vi "Configure ExecutionView Manager.vi"(8 "error in":errorcluster) -> (0 "error out":errorcluster)   [LabVIEW 2025, in "Config Tool.lvlib"]
doc: "This VI configures the Connections and Commands for the ExecutionView Manager."
uses:
  Control Globals.vi
  Config Tool.lvlib
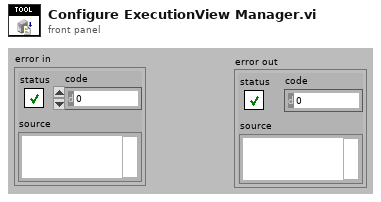
[diagram p1: front panel]
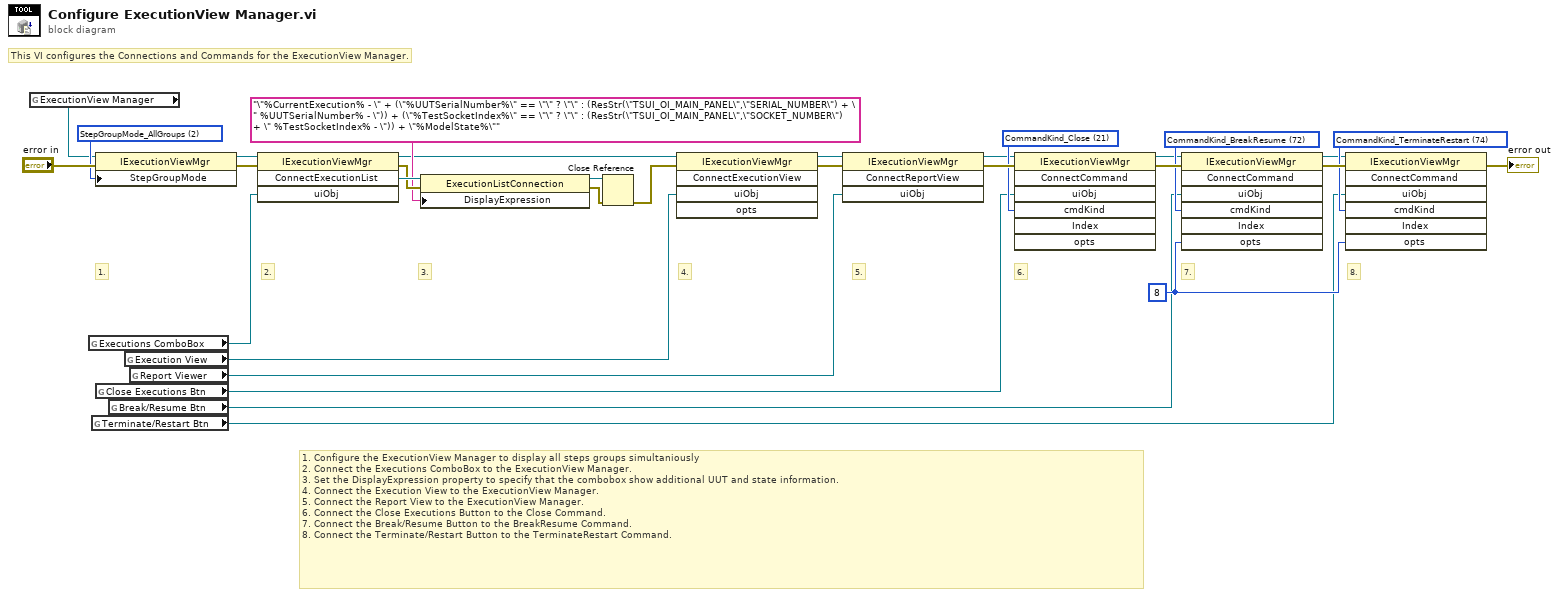
[diagram p0: block diagram]
diagram:
  w8 = 8 ("opts")
  w17 = 2 items=["StepGroupMode_OneGroup"=1, "StepGroupMode_AllGroups"=2] ("StepGroupMode")
  w20 = 74 items=["CommandKind_NotACommand"=0, "CommandKind_Container"=1, "CommandKind_Separator"=2, "CommandKind_Custom"=3, "CommandKind_OpenSequenceFile"=20, "CommandKind_Close"=21, "CommandKind_CloseAll"=22, "CommandKind_CloseCompletedExecutions"=23, "CommandKind_OpenWorkspaceBrowser"=24, "CommandKind_Login"=25, "CommandKind_Logout"=26, "CommandKind_LoginLogout"=27, "CommandKind_UnloadAllModules"=28, "CommandKind_MRUFile"=29, "CommandKind_Exit"=30, "CommandKind_Restart"=40, "CommandKind_RunEntryPoint"=41, "CommandKind_RunEntryPointOnSelectedSteps"=42, "CommandKind_LoopEntryPointOnSelectedSteps"=43, "CommandKind_RunCurrentSequence"=44, "CommandKind_RunSpecificSequence"=45, "CommandKind_RunSelectedSteps"=46, "CommandKind_RunSelectedStepsUsingEntryPointsSubmenu"=47, "CommandKind_LoopOnSelectedSteps"=48, "CommandKind_LoopOnSelectedStepsUsingEntryPointsSubmenu"=49, "CommandKind_BreakOnFirstStep"=50, "CommandKind_BreakOnStepFailure"=51, "CommandKind_BreakOnSequenceFailure"=52, "CommandKind_TracingEnabled"=53, "CommandKind_ToggleBreakpoint"=60, "CommandKind_SetRunModeSubmenu"=61, "CommandKind_RunModeForcePass"=62, "CommandKind_RunModeForceFail"=63, "CommandKind_RunModeSkip"=64, "CommandKind_RunModeNormal"=65, "CommandKind_Resume"=66, "CommandKind_StepInto"=67, "CommandKind_StepOver"=68, "CommandKind_StepOut"=69, "CommandKind_SetNextStep"=70, "CommandKind_Break"=71, "CommandKind_BreakResume"=72, "CommandKind_Terminate"=73, "CommandKind_TerminateRestart"=74, "CommandKind_Abort"=75, "CommandKind_BreakAll"=76, "CommandKind_TerminateAll"=77, "CommandKind_AbortAll"=78, "CommandKind_ResumeAll"=79, "CommandKind_DisplayBreakpointsAndWatchExpressions"=80, "CommandKind_DisplayBreakpointSettings"=81, "CommandKind_BreakpointSubmenu"=85, "CommandKind_ConfigureAdapters"=90, "CommandKind_ConfigureStationOptions"=91, "CommandKind_ConfigureSearchDirectories"=92, "CommandKind_ConfigureExternalViewers"=93, "CommandKind_ToolItem"=100, "CommandKind_CustomizeTools"=101, "CommandKind_ExecutionEntryPointInsertionMarker"=110, "CommandKind_ExecutionEntryPointDefaultMenuInsertionMarker"=111, "CommandKind_ConfigurationEntryPointInsertionMarker"=112, "CommandKind_ConfigurationEntryPointDefaultMenuInsertionMarker"=113, "CommandKind_DefaultFileMenu_Set"=120, "CommandKind_DefaultExecuteMenu_Set"=121, "CommandKind_DefaultDebugMenu_Set"=123, "CommandKind_DefaultConfigureMenu_Set"=124, "CommandKind_DefaultToolsMenu_Set"=125, "CommandKind_DefaultSequenceViewContextMenu_Set"=126, "CommandKind_DefaultListBarContextMenu_Set"=127, "CommandKind_MRUFiles_Set"=140, "CommandKind_ExecutionEntryPoints_Set"=141, "CommandKind_RunSequences_Set"=142, "CommandKind_RunSelectedStepsUsingEntryPoints_Set"=143, "CommandKind_LoopOnSelectedStepsUsingEntryPoints_Set"=144, "CommandKind_ConfigurationEntryPoints_Set"=145, "CommandKind_Tools_Set"=146] ("cmdKind")
  w21 = 72 items=["CommandKind_NotACommand"=0, "CommandKind_Container"=1, "CommandKind_Separator"=2, "CommandKind_Custom"=3, "CommandKind_OpenSequenceFile"=20, "CommandKind_Close"=21, "CommandKind_CloseAll"=22, "CommandKind_CloseCompletedExecutions"=23, "CommandKind_OpenWorkspaceBrowser"=24, "CommandKind_Login"=25, "CommandKind_Logout"=26, "CommandKind_LoginLogout"=27, "CommandKind_UnloadAllModules"=28, "CommandKind_MRUFile"=29, "CommandKind_Exit"=30, "CommandKind_Restart"=40, "CommandKind_RunEntryPoint"=41, "CommandKind_RunEntryPointOnSelectedSteps"=42, "CommandKind_LoopEntryPointOnSelectedSteps"=43, "CommandKind_RunCurrentSequence"=44, "CommandKind_RunSpecificSequence"=45, "CommandKind_RunSelectedSteps"=46, "CommandKind_RunSelectedStepsUsingEntryPointsSubmenu"=47, "CommandKind_LoopOnSelectedSteps"=48, "CommandKind_LoopOnSelectedStepsUsingEntryPointsSubmenu"=49, "CommandKind_BreakOnFirstStep"=50, "CommandKind_BreakOnStepFailure"=51, "CommandKind_BreakOnSequenceFailure"=52, "CommandKind_TracingEnabled"=53, "CommandKind_ToggleBreakpoint"=60, "CommandKind_SetRunModeSubmenu"=61, "CommandKind_RunModeForcePass"=62, "CommandKind_RunModeForceFail"=63, "CommandKind_RunModeSkip"=64, "CommandKind_RunModeNormal"=65, "CommandKind_Resume"=66, "CommandKind_StepInto"=67, "CommandKind_StepOver"=68, "CommandKind_StepOut"=69, "CommandKind_SetNextStep"=70, "CommandKind_Break"=71, "CommandKind_BreakResume"=72, "CommandKind_Terminate"=73, "CommandKind_TerminateRestart"=74, "CommandKind_Abort"=75, "CommandKind_BreakAll"=76, "CommandKind_TerminateAll"=77, "CommandKind_AbortAll"=78, "CommandKind_ResumeAll"=79, "CommandKind_DisplayBreakpointsAndWatchExpressions"=80, "CommandKind_DisplayBreakpointSettings"=81, "CommandKind_BreakpointSubmenu"=85, "CommandKind_ConfigureAdapters"=90, "CommandKind_ConfigureStationOptions"=91, "CommandKind_ConfigureSearchDirectories"=92, "CommandKind_ConfigureExternalViewers"=93, "CommandKind_ToolItem"=100, "CommandKind_CustomizeTools"=101, "CommandKind_ExecutionEntryPointInsertionMarker"=110, "CommandKind_ExecutionEntryPointDefaultMenuInsertionMarker"=111, "CommandKind_ConfigurationEntryPointInsertionMarker"=112, "CommandKind_ConfigurationEntryPointDefaultMenuInsertionMarker"=113, "CommandKind_DefaultFileMenu_Set"=120, "CommandKind_DefaultExecuteMenu_Set"=121, "CommandKind_DefaultDebugMenu_Set"=123, "CommandKind_DefaultConfigureMenu_Set"=124, "CommandKind_DefaultToolsMenu_Set"=125, "CommandKind_DefaultSequenceViewContextMenu_Set"=126, "CommandKind_DefaultListBarContextMenu_Set"=127, "CommandKind_MRUFiles_Set"=140, "CommandKind_ExecutionEntryPoints_Set"=141, "CommandKind_RunSequences_Set"=142, "CommandKind_RunSelectedStepsUsingEntryPoints_Set"=143, "CommandKind_LoopOnSelectedStepsUsingEntryPoints_Set"=144, "CommandKind_ConfigurationEntryPoints_Set"=145, "CommandKind_Tools_Set"=146] ("cmdKind")
  w22 = 21 items=["CommandKind_NotACommand"=0, "CommandKind_Container"=1, "CommandKind_Separator"=2, "CommandKind_Custom"=3, "CommandKind_OpenSequenceFile"=20, "CommandKind_Close"=21, "CommandKind_CloseAll"=22, "CommandKind_CloseCompletedExecutions"=23, "CommandKind_OpenWorkspaceBrowser"=24, "CommandKind_Login"=25, "CommandKind_Logout"=26, "CommandKind_LoginLogout"=27, "CommandKind_UnloadAllModules"=28, "CommandKind_MRUFile"=29, "CommandKind_Exit"=30, "CommandKind_Restart"=40, "CommandKind_RunEntryPoint"=41, "CommandKind_RunEntryPointOnSelectedSteps"=42, "CommandKind_LoopEntryPointOnSelectedSteps"=43, "CommandKind_RunCurrentSequence"=44, "CommandKind_RunSpecificSequence"=45, "CommandKind_RunSelectedSteps"=46, "CommandKind_RunSelectedStepsUsingEntryPointsSubmenu"=47, "CommandKind_LoopOnSelectedSteps"=48, "CommandKind_LoopOnSelectedStepsUsingEntryPointsSubmenu"=49, "CommandKind_BreakOnFirstStep"=50, "CommandKind_BreakOnStepFailure"=51, "CommandKind_BreakOnSequenceFailure"=52, "CommandKind_TracingEnabled"=53, "CommandKind_ToggleBreakpoint"=60, "CommandKind_SetRunModeSubmenu"=61, "CommandKind_RunModeForcePass"=62, "CommandKind_RunModeForceFail"=63, "CommandKind_RunModeSkip"=64, "CommandKind_RunModeNormal"=65, "CommandKind_Resume"=66, "CommandKind_StepInto"=67, "CommandKind_StepOver"=68, "CommandKind_StepOut"=69, "CommandKind_SetNextStep"=70, "CommandKind_Break"=71, "CommandKind_BreakResume"=72, "CommandKind_Terminate"=73, "CommandKind_TerminateRestart"=74, "CommandKind_Abort"=75, "CommandKind_BreakAll"=76, "CommandKind_TerminateAll"=77, "CommandKind_AbortAll"=78, "CommandKind_ResumeAll"=79, "CommandKind_DisplayBreakpointsAndWatchExpressions"=80, "CommandKind_DisplayBreakpointSettings"=81, "CommandKind_BreakpointSubmenu"=85, "CommandKind_ConfigureAdapters"=90, "CommandKind_ConfigureStationOptions"=91, "CommandKind_ConfigureSearchDirectories"=92, "CommandKind_ConfigureExternalViewers"=93, "CommandKind_ToolItem"=100, "CommandKind_CustomizeTools"=101, "CommandKind_ExecutionEntryPointInsertionMarker"=110, "CommandKind_ExecutionEntryPointDefaultMenuInsertionMarker"=111, "CommandKind_ConfigurationEntryPointInsertionMarker"=112, "CommandKind_ConfigurationEntryPointDefaultMenuInsertionMarker"=113, "CommandKind_DefaultFileMenu_Set"=120, "CommandKind_DefaultExecuteMenu_Set"=121, "CommandKind_DefaultDebugMenu_Set"=123, "CommandKind_DefaultConfigureMenu_Set"=124, "CommandKind_DefaultToolsMenu_Set"=125, "CommandKind_DefaultSequenceViewContextMenu_Set"=126, "CommandKind_DefaultListBarContextMenu_Set"=127, "CommandKind_MRUFiles_Set"=140, "CommandKind_ExecutionEntryPoints_Set"=141, "CommandKind_RunSequences_Set"=142, "CommandKind_RunSelectedStepsUsingEntryPoints_Set"=143, "CommandKind_LoopOnSelectedStepsUsingEntryPoints_Set"=144, "CommandKind_ConfigurationEntryPoints_Set"=145, "CommandKind_Tools_Set"=146] ("cmdKind")
  # "8."
  # "7."
  # "6."
  # "5."
  # "4."
  # "3."
  # "2."
  # "1."
  # "1. Configure the ExecutionView Manager to display all steps groups simultaniously\n2. Connect the Executions ComboBox to the ExecutionView Manager. \n3. Set the DisplayExpression property to specify that the combobox show additional UUT and state information.\n4. Connect the Execution View to the ExecutionView Manager.\n5. Connect the Report View to the ExecutionView Manager.\n6. Connect the Close Executions Button to the Close Command.\n7. Connect the Break/Resume Button to the BreakResume Command. \n8. Connect the Terminate/Restart Button to the TerminateRestart Command."
  # "This VI configures the Connections and Commands for the ExecutionView Manager."
  n1 = global read "Control Globals.vi" "ExecutionView Manager"() -> (w7:refnum<k7>)
  n2 = global read "Control Globals.vi" "Executions ComboBox"() -> (w6:refnum<k7>)
  n3 = global read "Control Globals.vi" "Terminate/Restart Btn"() -> (w1:refnum<k7>)
  n4 = property class="IExecutionViewMgr"(reference=w7, error in="error in", "StepGroupMode"=w17) -> (reference out=w18:refnum<k7>, error out=w19:errorcluster)
  n5 = global read "Control Globals.vi" "Close Executions Btn"() -> (w3:refnum<k7>)
  n6 = global read "Control Globals.vi" "Break/Resume Btn"() -> (w2:refnum<k7>)
  n7 = global read "Control Globals.vi" "Execution View"() -> (w5:refnum<k7>)
  n8 = global read "Control Globals.vi" "Report Viewer"() -> (w4:refnum<k7>)
  n9 = invoke class="IExecutionViewMgr" method="ConnectExecutionList"(reference=w18, error in=w19, "uiObj"=w6) -> (reference out=w13:refnum<k7>, error out=w24:errorcluster, "ConnectExecutionList"=w25:refnum<k7>)  [unwired: 1 in, 1 out]
  n10 = property class="ExecutionListConnection"(reference=w25, error in=w24, "DisplayExpression"="\"%CurrentExecution% - \" + (\"%UUTSerialNumber%\" == \"\" ? \"\" : (ResStr(\"TSUI_OI_MAIN_PANEL\",\"SERIAL_NUMBER\") + \" %UUTSerialNumber% - \")) + (\"%TestSocketIndex%\" == \"\" ? \"\" : (ResStr(\"TSUI_OI_MAIN_PANEL\",\"SOCKET_NUMBER\") + \" %TestSocketIndex% - \")) + \"%ModelState%\"") -> (reference out=w14:refnum<k7>, error out=w15:errorcluster)
  n11 = Close Reference(reference=w14, error in (no error)=w15) -> (error out=w16:errorcluster)
  n12 = invoke class="IExecutionViewMgr" method="ConnectExecutionView"(reference=w13, error in=w16, "uiObj"=w5) -> (reference out=w9:refnum<k7>, error out=w26:errorcluster)  [unwired: 2 in, 3 out]
  n13 = invoke class="IExecutionViewMgr" method="ConnectReportView"(reference=w9, error in=w26, "uiObj"=w4) -> (reference out=w10:refnum<k7>, error out=w27:errorcluster)  [unwired: 1 in, 2 out]
  n14 = invoke class="IExecutionViewMgr" method="ConnectCommand"(reference=w10, error in=w27, "uiObj"=w3, "cmdKind"=w22) -> (reference out=w11:refnum<k7>, error out=w28:errorcluster)  [unwired: 3 in, 5 out]
  n15 = invoke class="IExecutionViewMgr" method="ConnectCommand"(reference=w11, error in=w28, "uiObj"=w2, "cmdKind"=w21, "opts"=w8) -> (reference out=w12:refnum<k7>, error out=w29:errorcluster)  [unwired: 2 in, 5 out]
  n16 = invoke class="IExecutionViewMgr" method="ConnectCommand"(reference=w12, error in=w29, "uiObj"=w1, "cmdKind"=w20, "opts"=w8) -> (error out=→"error out":errorcluster)  [unwired: 2 in, 6 out]
